vi "Tracepoint_ServerError.vi"(8 "error in (no error)":errorcluster, 9 "String":string, 10 "Error":bool, 11 "Qbus":refnum<class "Qbus.lvclass">) -> (0 "error out":errorcluster)   [LabVIEW 2017, in "OPCUAClient.lvlib"]
uses:
  <vilib>/addons/InsightCM/Devices/Shared/Common/OPCUAClient/OPCUAClient.lvlib
  <vilib>/addons/Qbus/Qbus.lvclass
  <vilib>/addons/TraceLogger/TraceLogger.lvlib
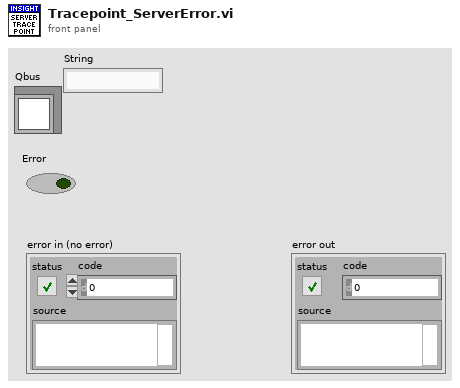
[diagram p1: front panel]
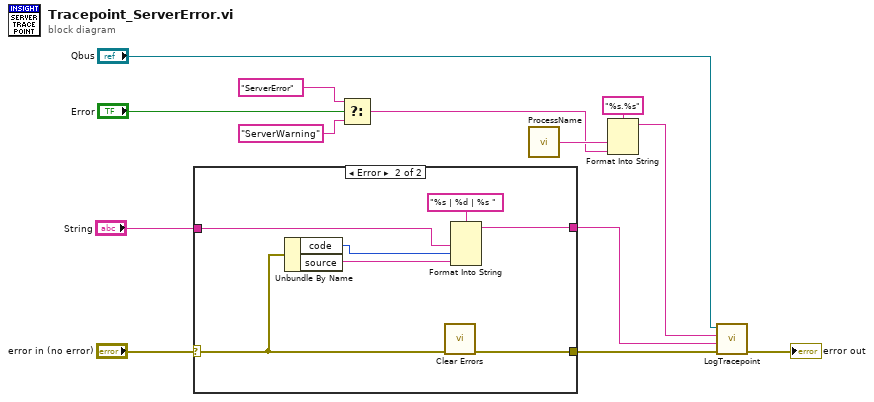
[diagram p0: block diagram]
diagram:
  n1 = case shown="Error" "error in (no error)" {
    selector: "error in (no error)" -> [w15 w19]
    tunnel: [w15 w22] -> w4
    tunnel: [w14 w20] -> w3
    tunnel: "String" -> [w14 w16]
    frame No Error {
    }
    frame Error {
      n2 = Unbundle By Name(w19) -> ("code"=w18:i32, "source"=w17:string)
      n3 = call <vilib>:"Clear Errors.vi"("error in (no error)"=w19) -> ("error out"=w22:errorcluster)  [unwired: 5 in, 1 out]
      n4 = Format Into String(format string="%s | %d | %s ", w16, w18, w17) -> (resulting string=w20:string)  [unwired: 2 in, 1 out]
    }
  }
  n5 = Select(t="ServerError" ("tracepoint"), s="Error", f="ServerWarning" ("tracepoint")) -> (s? t:f=w6:string)
  n6 = call <vilib>:"ProcessName.vi"() -> ("process name"=w10:string)  [unwired: 5 in]
  n7 = Format Into String(format string="%s.%s", w10, w6) -> (resulting string=w5:string)  [unwired: 2 in, 1 out]
  n8 = call <vilib>:"LogTracepoint.vi"("error in (no error)"=w4, "log string"=w3, "tracepoint"=w5, "qbus in"="Qbus") -> ("error out"=→"error out":errorcluster)  [unwired: 6 in, 1 out]
